vi "Populate Document Elements.vi"(8 "error in (no error)":errorcluster, 11 "xwpfDocument in":refnum<class "xwpfDocument.lvclass">) -> (0 "error out":errorcluster, 3 "xwpfDocument out":refnum<class "xwpfDocument.lvclass">)   [LabVIEW 2017, in "Word_Specific.lvlib" / "xwpfDocument.lvclass"]
uses:
  xwpfDocument.lvclass
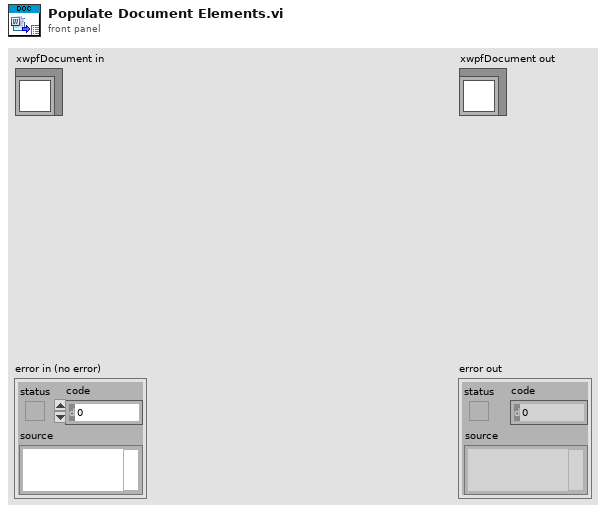
[diagram p1: front panel]
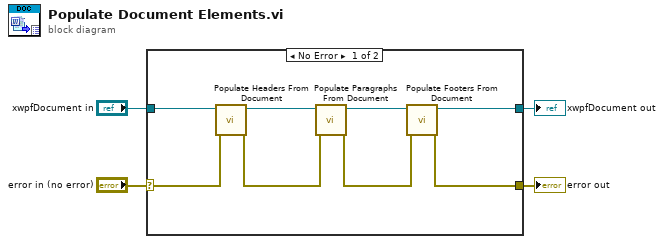
[diagram p0: block diagram]
diagram:
  n1 = case shown="No Error" "error in (no error)" {
    selector: "error in (no error)" -> [w8 w14]
    tunnel: [w5 w14] -> w3
    tunnel: [w7 w13] -> w1
    tunnel: "xwpfDocument in" -> [w11 w13]
    frame No Error {
      n2 = call "Populate Headers From Document.vi"("error in (no error)"=w8, "xwpfDocument in"=w11) -> ("error out"=w9:errorcluster, "xwpfDocument out"=w12:refnum<class "xwpfDocument.lvclass">)  [unwired: 8 in]
      n3 = call "Populate Paragraphs From Document.vi"("error in (no error)"=w9, "xwpfDocument in"=w12) -> ("error out"=w6:errorcluster, "xwpfDocument out"=w10:refnum<class "xwpfDocument.lvclass">)  [unwired: 8 in]
      n4 = call "Populate Footers From Document.vi"("error in (no error)"=w6, "xwpfDocument in"=w10) -> ("error out"=w5:errorcluster, "xwpfDocument out"=w7:refnum<class "xwpfDocument.lvclass">)  [unwired: 8 in]
    }
    frame Error {
    }
  }
  "error out" <- w3
  "xwpfDocument out" <- w1
